vi "Drop Message.vi"(11 "Channel Message in":refnum<class "Channel Message.lvclass">) -> (3 "Channel Message out":refnum<class "Channel Message.lvclass">)   [LabVIEW 2020, in "Channel Message.lvclass"]
doc: "This method defines what a message does if it is in the Messenger Channel when the channel is aborted. At this point, the reader loop has shut down, so it will never read the message.\n\nBy default, this method does nothing. Override this method in a child class ONLY if this is a message where the sender needs some sort of acknowledgement signal or if you need to release some resource that is being carried by the message. For example, you might have a message whose job was to transfer ownership of a refnum from the writer to the reader. Since the reader will never know about that transfer, the Drop Message override can be used to release the refnum."
uses:
  <vilib>/ChannelSupport/Channel Message/Channel Message.lvclass
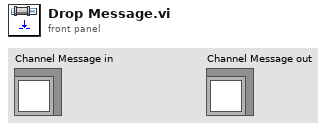
[diagram p1: front panel]
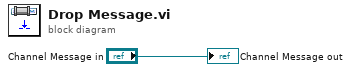
[diagram p0: block diagram]
diagram:
  "Channel Message out" <- "Channel Message in"
